vi "Set Speed millliGAT.vi"() -> ()   [LabVIEW 2018, in "VICI M6 M50 Party Mode.lvlib"]
uses:
  VICI M6 M50 Party Mode.lvlib
  Settings Cluster.ctl
panel:
  in  "VICI Settings":T1
  in  "Flow Rate (mL/min)":dbl format="%.2f"
  out "x/y":dbl
  out "concatenated string":string
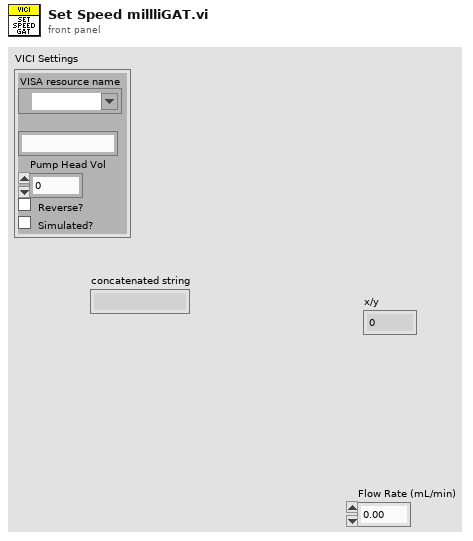
[diagram p1: front panel]
types:
  T1 = typedef "VICI M6 M50 Party Mode.lvlib/Settings Cluster.ctl" = cluster{"VISA resource name":refnum<visa-resource-name>, "Pump ID":string, "Pump Head Vol":dbl, "Reverse?":bool, "Simulated?":bool}
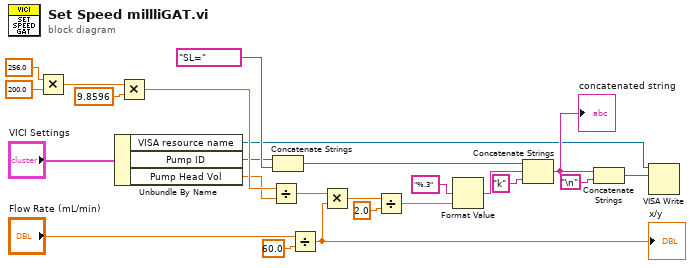
[diagram p0: block diagram]
diagram:
  n1 = Multiply(x=256.0, y=200.0) -> (x*y=w21:dbl)
  n2 = Unbundle By Name("VICI Settings") -> ("VISA resource name"=w3:refnum<visa-resource-name>, "Pump ID"=w2:string, "Pump Head Vol"=w1:dbl)
  n3 = Multiply(x=w21, y=9.8596) -> (x*y=w10:dbl)
  n4 = Divide(x=w10, y=w1) -> (x/y=w11:dbl)
  n5 = Concatenate Strings(w2, "SL=") -> (w24:string)
  n6 = Divide(x="Flow Rate (mL/min)", y=60.0) -> (x/y=w12:dbl)
  "x/y" <- w12
  n7 = Multiply(x=w11, y=w12) -> (x*y=w8:dbl)
  n8 = Divide(x=w8, y=2.0) -> (x/y=w7:dbl)
  n9 = Format Value(format string="%.3", value (0)=w7) -> (output string=w17:string)  [unwired: 1 in]
  n10 = Concatenate Strings(w24, w17, "k" ("string")) -> (w16:string)
  "concatenated string" <- w16
  n11 = Concatenate Strings(w16, "\n") -> (w14:string)
  n12 = VISA Write(VISA resource name=w3, write buffer=w14) -> ()  [unwired: 1 in, 3 out]
